vi "Programmatically populate tree control.vi"() -> ()   [LabVIEW 2019]
uses:
  <vilib>/httpClient/POSTBuffer.vi
  <vilib>/httpClient/LabVIEWHTTPClient.lvlib
panel:
  in  "TreeDone":string(tree)
  in  "Asc?":bool
  in  "stop":bool
  out "Double Click":string
  in  "TreeRun":string(tree)
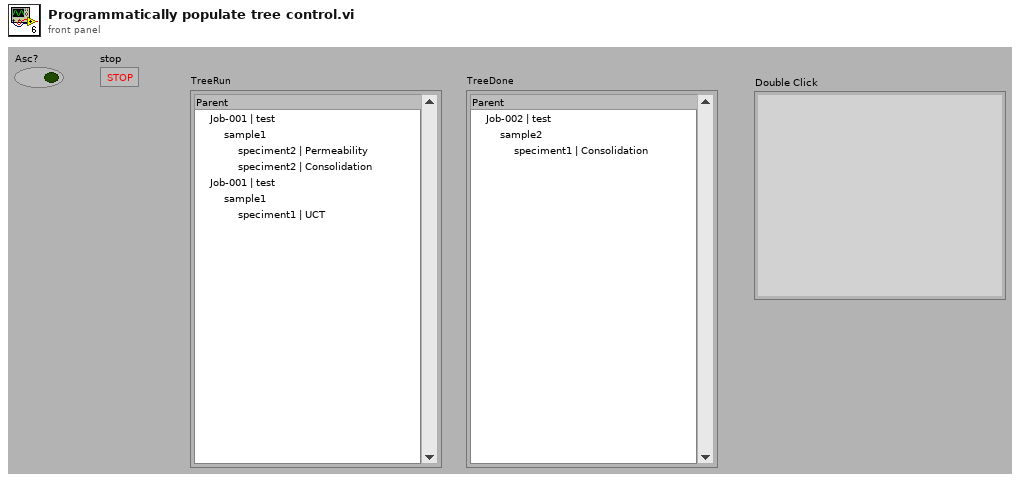
[diagram p1: front panel]
types:
  T1 = typedef "LabVIEWHTTPClient.lvlib/ClientHandle.ctl" = refnum<k1>
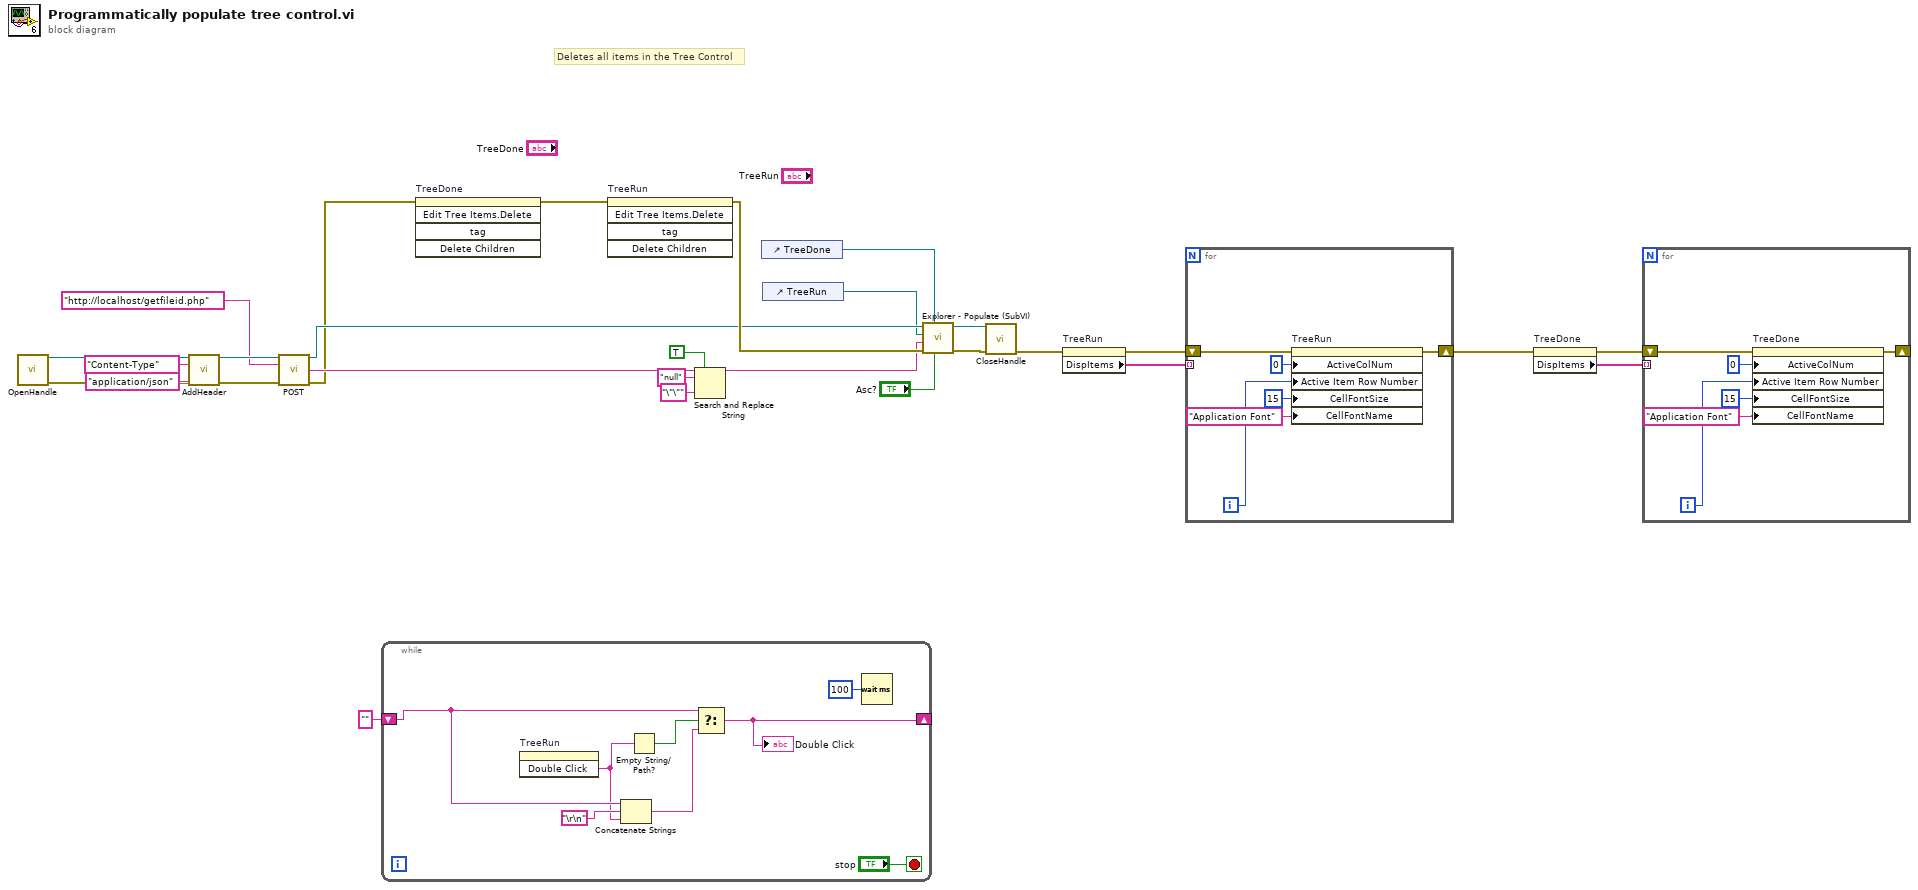
[diagram p0: block diagram]
diagram:
  # "Deletes all items in the Tree Control"
  n1 = call <vilib>:"OpenHandle.vi"() -> ("client handle out"=w24:T1, "error out"=w22:errorcluster)  [unwired: 14 in]
  n2 = call <vilib>:"AddHeader.vi"("client handle"=w24, "header"="Content-Type", "value"="application/json", "error in (no error)"=w22) -> ("client handle out"=w25:T1, "error out"=w23:errorcluster)  [unwired: 10 in]
  n3 = call-poly <vilib>:"POST.vi"("client handle"=w25, "url"="http://localhost/getfileid.php", "error in (no error)"=w23) -> ("client handle out"=w11:T1, "body"=w17:string, "error out"=w7:errorcluster)  [unwired: 9 in, 1 out]
  n4 = while {
    shift-right: [w29] -> _
    shift-left: "" -> [w33]
    stop <- "stop" stop-if-true
    n5 = invoke on="TreeRun" class="Tree (strict)" method="Double Click"() -> ("Double Click"=w31:string)  [unwired: 3 in, 2 out]
    n6 = Concatenate Strings(w33, "\r\n", w31) -> (w30:string)
    n7 = Empty String/Path?(string/path=w31) -> (empty?=w34:bool)
    n8 = Select(t=w33, s=w34, f=w30) -> (s? t:f=w29:string)
    "Double Click" <- w29
    n9 = Wait (ms)(milliseconds to wait=u32 100) -> ()  [unwired: 1 out]
  }
  n10 = invoke on="TreeDone" class="Tree (strict)" method="Edit Tree Items.Delete"(error in=w7) -> (error out=w6:errorcluster)  [unwired: 4 in, 4 out]
  n11 = invoke on="TreeRun" class="Tree (strict)" method="Edit Tree Items.Delete"(error in=w6) -> (error out=w28:errorcluster)  [unwired: 4 in, 4 out]
  n12 = Search and Replace String(replace all?=TRUE ("replace all? (F)"), input string=w17, search string="null", replace string="\"\"" ("replace string (\"\")")) -> (result string=w16:string)  [unwired: 4 in, 3 out]
  n13 = control-ref of="TreeDone"() -> (w8:refnum<vi>)
  n14 = control-ref of="TreeRun"() -> (w10:refnum<vi>)
  n15 = call "Explorer - Populate (SubVI).vi"("Asc?"="Asc?", "TreeDone"=w8, "error in (no error)"=w28, "Test Data"=w16, "TreeRun"=w10, "RefIn"=w11) -> ("error out"=w13:errorcluster, "Refnum out"=w20:T1)  [unwired: 2 in, 2 out]
  n16 = call <vilib>:"CloseHandle.vi"("client handle"=w20, "error in (no error)"=w13) -> ("error out"=w12:errorcluster)  [unwired: 13 in]
  n17 = property on="TreeRun" class="Tree (strict)"(error in=w12) -> (error out=w5:errorcluster, "DispItems"=w2:string[])  [unwired: 1 in, 1 out]
  n18 = for {
    shift-right: [w37] -> w4
    shift-left: w5 -> [w42]
    tunnel: w2 -> [_] mode=indexing
    i -> [w39]
    n19 = property on="TreeRun" class="Tree (strict)"(error in=w42, "ActiveColNum"=0 ("Active Item:Row Number"), "Active Item Row Number"=w39, "CellFontSize"=u32 15 ("Active Cell:Cell Font:Size"), "CellFontName"="Application Font" ("Active Cell:Cell Font:Name")) -> (error out=w37:errorcluster)  [unwired: 1 in, 1 out]
  }
  n20 = property on="TreeDone" class="Tree (strict)"(error in=w4) -> (error out=w3:errorcluster, "DispItems"=w1:string[])  [unwired: 1 in, 1 out]
  n21 = for {
    shift-right: [w47] -> _
    shift-left: w3 -> [w48]
    tunnel: w1 -> [_] mode=indexing
    i -> [w45]
    n22 = property on="TreeDone" class="Tree (strict)"(error in=w48, "ActiveColNum"=0 ("Active Item:Row Number"), "Active Item Row Number"=w45, "CellFontSize"=u32 15 ("Active Cell:Cell Font:Size"), "CellFontName"="Application Font" ("Active Cell:Cell Font:Name")) -> (error out=w47:errorcluster)  [unwired: 1 in, 1 out]
  }
